vi "Query.vi"(8 "error in (no error)":errorcluster, 11 "UI VISA Terminal in":refnum<class "UI VISA Terminal.lvclass">) -> (0 "error out":errorcluster, 3 "UI VISA Terminal out":refnum<class "UI VISA Terminal.lvclass">)   [LabVIEW 2025, in "UI VISA Terminal.lvlib" / "UI VISA Terminal.lvclass"]
uses:
  UI VISA Terminal.lvclass
  UI VISA Terminal.lvclass/UI VISA Terminal.ctl
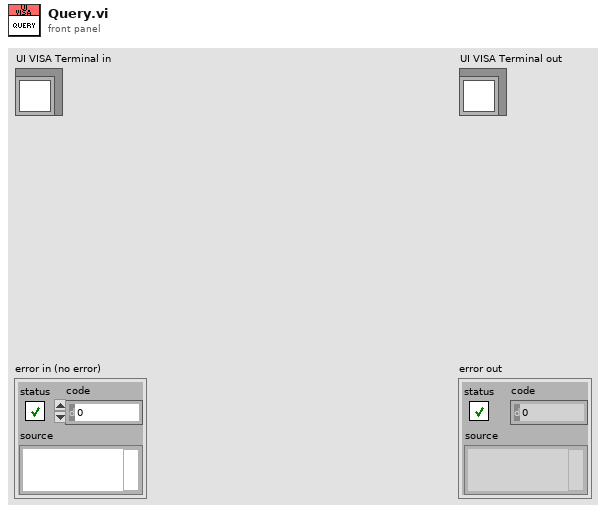
[diagram p1: front panel]
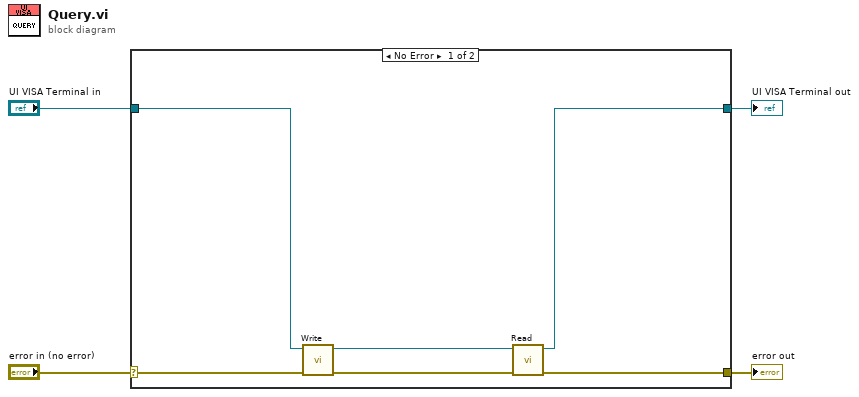
[diagram p0: block diagram]
diagram:
  n1 = case shown="No Error" "error in (no error)" {
    selector: "error in (no error)" -> [w10 w12]
    tunnel: [w8 w12] -> w3
    tunnel: [w5 w11] -> w1
    tunnel: "UI VISA Terminal in" -> [w7 w11]
    frame No Error {
      n2 = call-dynamic "Write.vi"("error in (no error)"=w10, "UI VISA Terminal in"=w7) -> ("error out"=w9:errorcluster, "UI VISA Terminal out"=w6:refnum<class "UI VISA Terminal.lvclass">)  [unwired: 8 in]
      n3 = call-dynamic "Read.vi"("error in (no error)"=w9, "UI VISA Terminal in"=w6) -> ("error out"=w8:errorcluster, "UI VISA Terminal out"=w5:refnum<class "UI VISA Terminal.lvclass">)  [unwired: 8 in]
    }
    frame Error {
    }
  }
  "error out" <- w3
  "UI VISA Terminal out" <- w1
